vi "Accept.vi"(8 "Error in (no error)":errorcluster, 10 "Log in":T1 {"Priority" items=["EMERGENCY", "ALERT", "CRITICAL", "ERROR", "WARNING", "NOTICE", "INFO", "DEBUG"]}, 11 "LogFilterSupress in":refnum<class "LogFilterSupress.lvclass">) -> (0 "Error out":errorcluster, 2 "Accept":bool, 3 "LogFilterSupress out":refnum<class "LogFilterSupress.lvclass">)   [LabVIEW 2011, in "LogFilterSupress.lvclass"]
uses:
  LogFilterSupress.lvclass
  Log/LogCluster.ctl
  Log/PrioritiesRing.ctl
  LogFilterSupress.lvclass/LogFilterSupress.ctl
  Log/Log.lvclass
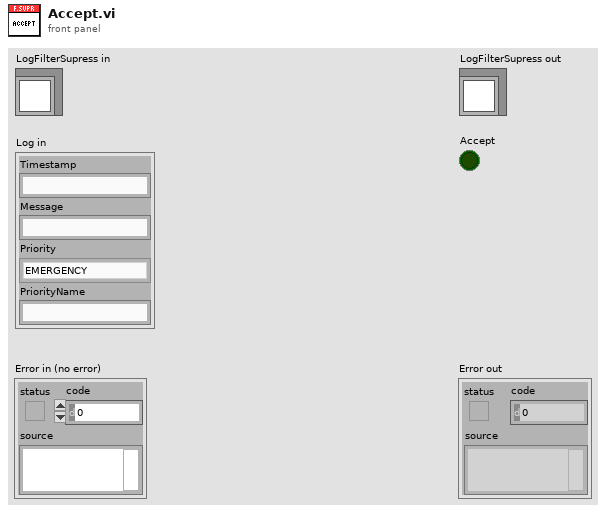
[diagram p1: front panel]
types:
  T1 = typedef "Log.lvclass/LogCluster.ctl" = cluster{"Timestamp":string, "Message":string, "Priority":T2, "PriorityName":string}
  T2 = typedef "Log.lvclass/PrioritiesRing.ctl" = u32
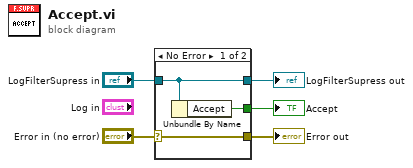
[diagram p0: block diagram]
diagram:
  n1 = case shown="No Error" "Error in (no error)" {
    selector: "Error in (no error)" -> [w8 w10]
    tunnel: [w8 w10] -> w4
    tunnel: [w7 w9] -> w2
    tunnel: "LogFilterSupress in" -> [w7 w9]
    tunnel: [w6 _] -> w1
    frame No Error {
      n2 = Unbundle By Name(w7) -> ("Accept"=w6:bool)
    }
    frame Error {
    }
  }
  "Error out" <- w4
  "LogFilterSupress out" <- w2
  "Accept" <- w1
